vi "Write.vi"   [LabVIEW 2009, in "MicroDAQ.lvlib"]
doc: "Writes samples to output channels. This VI is polimorphic and will adapt to source"
uses:
  <instrlib>/MicroDAQ/MicroDAQ.lvlib
  <instrlib>/MicroDAQ/Channel/Analog Output/Analog output.lvclass
  <instrlib>/MicroDAQ/Channel/Digital output/Digital output.lvclass
  <instrlib>/MicroDAQ/Channel/DSP/DSP.lvclass
  <instrlib>/MicroDAQ/Channel/PWM/PWM.lvclass
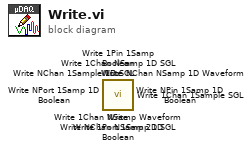
[diagram p0: block diagram]
diagram:
  n1 = call <instrlib>:"Write.vi"() -> ()  [unwired: 10 in, 2 out]
  n2 = call <instrlib>:"Write.vi"() -> ()  [unwired: 10 in, 2 out]
  n3 = call <instrlib>:"Write NPort 1Samp 1D Boolean.vi"() -> ()  [unwired: 10 in, 2 out]
  n4 = call <instrlib>:"Write NPin 1Samp 1D Boolean.vi"() -> ()  [unwired: 10 in, 2 out]
  n5 = call <instrlib>:"Write 1Port 1Samp 1D Boolean.vi"() -> ()  [unwired: 10 in, 2 out]
  n6 = call <instrlib>:"Write 1Pin 1Samp Boolean.vi"() -> ()  [unwired: 10 in, 2 out]
  n7 = call <instrlib>:"Write 1Chan NSamp Waveform.vi"() -> ()  [unwired: 10 in, 2 out]
  n8 = call <instrlib>:"Write NChan NSamp 1D Waveform.vi"() -> ()  [unwired: 10 in, 2 out]
  n9 = call <instrlib>:"Write NChan 1Sample 1D SGL.vi"() -> ()  [unwired: 10 in, 2 out]
  n10 = call <instrlib>:"Write 1Chan NSamp 1D SGL.vi"() -> ()  [unwired: 10 in, 2 out]
  n11 = call <instrlib>:"Write 1Chan 1Sample SGL.vi"() -> ()  [unwired: 10 in, 2 out]
  n12 = call <instrlib>:"Write NChan NSamp 2D SGL.vi"() -> ()  [unwired: 10 in, 2 out]
